vi "TCPWait.vi"(8 "error in":errorcluster, 11 "StructIn":T1) -> (0 "error out":errorcluster, 1 "Connected":bool, 2 "remote address":string, 3 "StructOut":T1)   [LabVIEW 2021, in "LibDan.lvlib"]
uses:
  LibDan.lvlib
  TerminalDef.ctl
  <vilib>/Utility/config.llb/Config Data RefNum.ctl
  <vilib>/Utility/config.llb/NI_LVConfig.lvlib
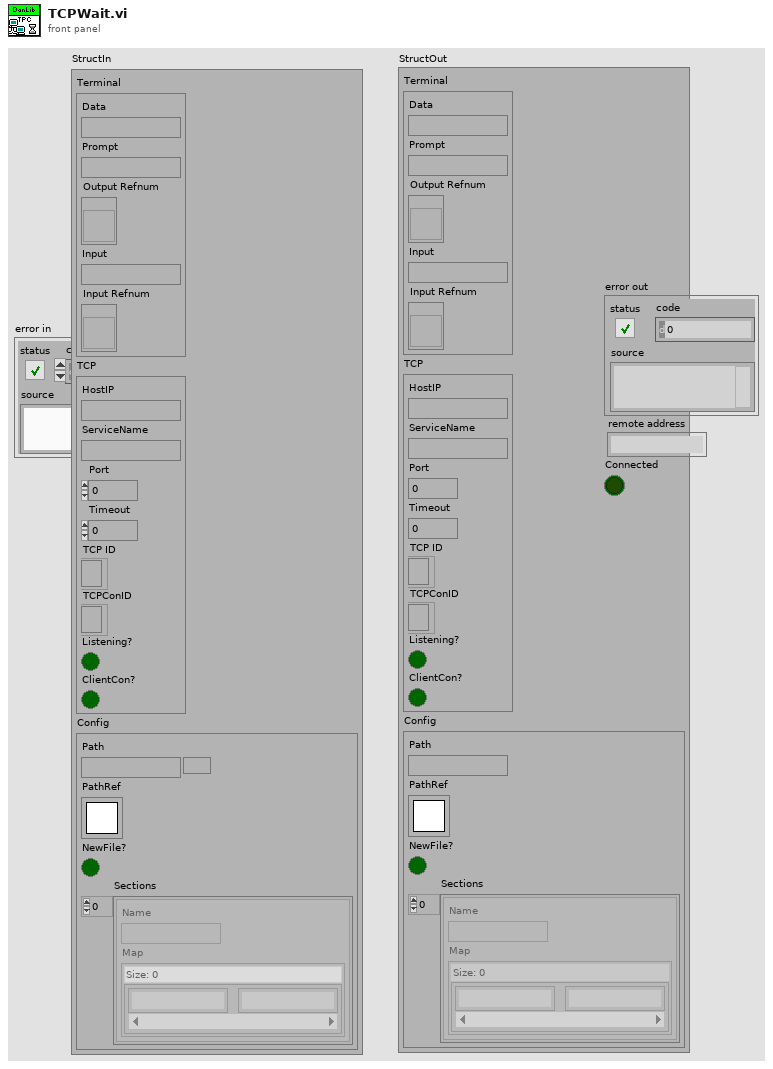
[diagram p1: front panel]
types:
  T1 = typedef "LibDan.lvlib/TerminalDef.ctl" = cluster{"Terminal":cluster{"Data":string, "Prompt":string, "Output Refnum":refnum<vi>, "Input":string, "Input Refnum":refnum<vi>}, "TCP":cluster{"HostIP":string, "ServiceName":string, "Port":u16, "Timeout":i32, "TCP ID":refnum<k5>, "TCPConID":refnum<k5>, "Listening?":bool, "ClientCon?":bool}, "Config":cluster{"Path":path, "PathRef":T2, "NewFile?":bool, "Sections":cluster{"Name":string, "Map":map{string, string}}[]}}
  T2 = typedef "NI_LVConfig.lvlib/Config Data RefNum.ctl" = refnum<k1>
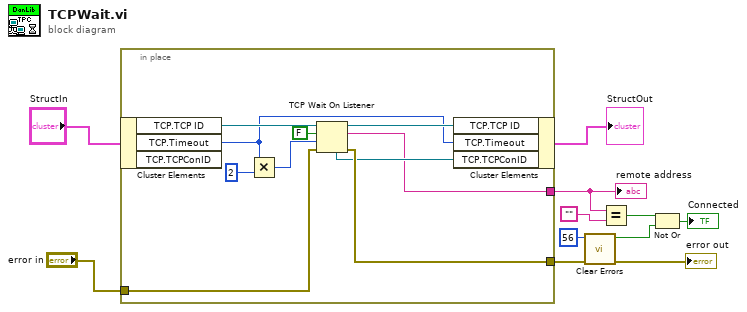
[diagram p0: block diagram]
diagram:
  n1 = in-place {
    in-place-border: "error in" -> [w21]
    in-place-border: [w19] -> w6
    in-place-border: [w14] -> w2
    n2 = in-place-cluster #1("StructIn") -> ("TCP.TCP ID"=w18:refnum<k5>, "TCP.Timeout"=w13:i32)  [unwired: 1 out]
    n3 = Multiply(x=w13, y=2) -> (x*y=w16:i32)
    n4 = TCP Wait On Listener(8:w21, 9:w16, 10:FALSE ("resolve remote address (T)"), 11:w18) -> (0:w19:errorcluster, 2:w14:string, 3:w20:refnum<k5>, 4:w15:refnum<k5>)  [unwired: 1 out]
    n5 = in-place-cluster #1("TCP.TCP ID"=w20, "TCP.Timeout"=w13, "TCP.TCPConID"=w15) -> (→"StructOut":T1)
  }
  "remote address" <- w2
  n6 = call <vilib>:"Clear Errors.vi"("error in (no error)"=w6, "specific error code to clear (0: all)"=56) -> ("error out"=→"error out":errorcluster, "specific error cleared?"=w1:bool)  [unwired: 4 in]
  n7 = Equal?(x=w2, y="") -> (x = y?=w4:bool)
  n8 = Not Or(1:w1, 2:w4) -> (0:→"Connected":bool)
